vi "EG_G5210 ReadCh.vi"(0 "VISA Rsrc":refnum<visa-resource-name>="SR530", 1 "StatusByteRef":refnum<vi>, 5 "Channel":T1(ring), 7 "Autoscale":bool, 9 "Check Status":bool=TRUE, 11 "error in (no error)":errorcluster, 12 "Ask Correction":bool, 13 "ShowStatMess":bool=TRUE caption="Show Status Message") -> (2 "Sensitivity":u16(ring)=13 items=["100 nV", "300 nV", "1 µV", "3 µV", "10 µV", "30 µV", "100µV", "300 µV", "1 mV", "3 mV", "10 mV", "30 mV", "100 mV", "300 mV", "1 V", "3 V"], 3 "Status Byte":bool[](array[boolean]), 4 "Ressource VISA Out":refnum<visa-resource-name>="GPIB0::8::INSTR", 6 "Outputs":dbl[](array[numeric]), 8 "Outputs %":dbl[](array[numeric]), 10 "Warning":bool, 14 "Ask Correction Out":bool, 15 "error out":errorcluster)   [LabVIEW 2010]
uses:
  <userlib>/EG_G 5210 LIA/ReadChStates.ctl
  <userlib>/EG_G 5210 LIA/ReadFunctions.ctl
panel:
  out "Input Mode":u16(ring) items=["Current 10E8 A/V", "Current 10E6 A/V", "Voltage"]
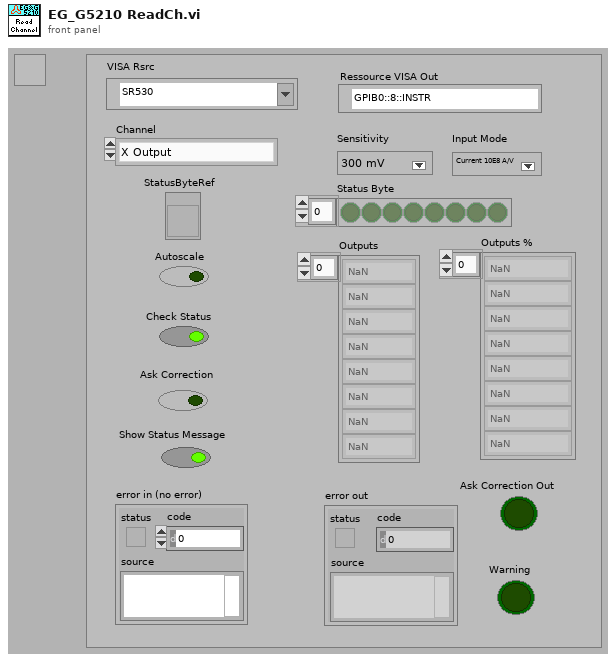
[diagram p1: front panel]
types:
  T1 = enum16{"X Output", "Y Output", "X and Y Output", "Mag", "Phase", "Mag & Phase", "X,Y,Mag & Phase", "Noise", "Aux In 1", "Aux In 2", "Aux In 3", "Aux In 4"}
  T2 = typedef "ReadChStates.ctl" = enum16{"Check Status", "Read Scale", "Read Ch"}
  T3 = typedef "ReadFunctions.ctl" = enum16{"Sensitivity", "Vernier Mode", "Main Filter", "Filter Mode", "Line Filter", "Ref Source", "Ref Mode", "Ref Phase", "Ref Frequency", "Output Filter", "Time Constant", "Dyn Reserve", "X Offset", "Y Offset", "Expand Mode", "Int Oscillator", "Oscillator Freq", "All params", "Overload Byte", "Trigger Mode", "Error"}
  T4 = typedef "LockInPar.ctl" = cluster{"Sensitivity":u16, "Vernier Mode":bool, "Vernier Value":i32, "Main Filter":u16, "Filter Freq (Hz)":dbl, "Filter Mode":u16, " Line Notch":u16, "Reference":u16, "Reference Mode":u16, "Ref Phase (°)":dbl, "Ref Freq (Hz)":dbl, "Output Filter":u16, "Time Constant":u16, "Dynamic Res.":u16, "X Offset":bool, "X Offset Val %":dbl, "Y Offset":bool, "Y Offset Val %":dbl, "Expand":bool, "Osc Amp. (mV rms)":i32, "Int Osc (Hz)":dbl, "Trigger Mode":u16, "Input Mode":u16, "Ovld Source":u16}
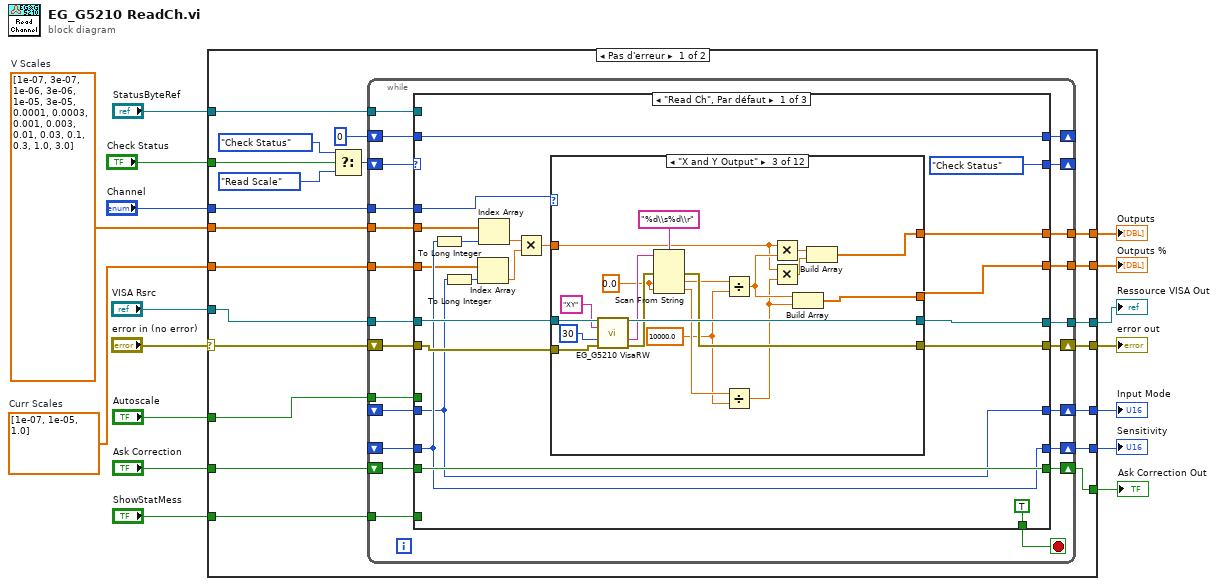
[diagram p0: block diagram]
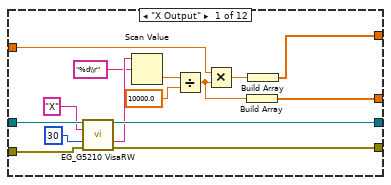
[diagram p2: hidden frame]
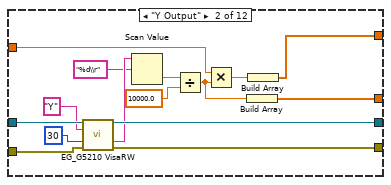
[diagram p3: hidden frame]
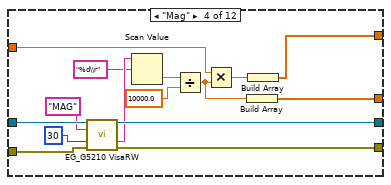
[diagram p4: hidden frame]
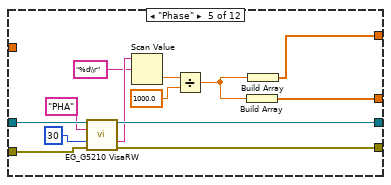
[diagram p5: hidden frame]
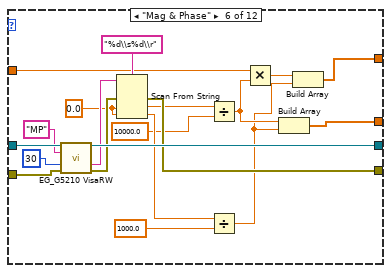
[diagram p6: hidden frame]
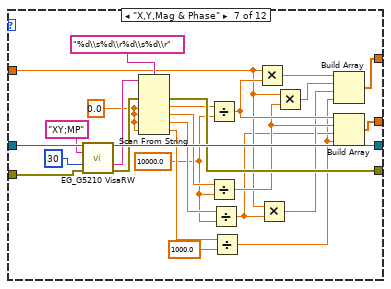
[diagram p7: hidden frame]
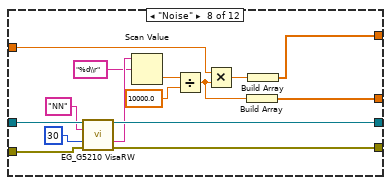
[diagram p8: hidden frame]
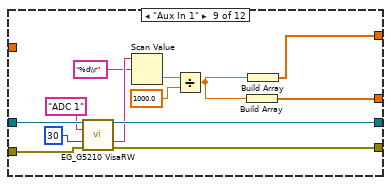
[diagram p9: hidden frame]
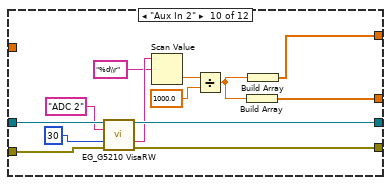
[diagram p10: hidden frame]
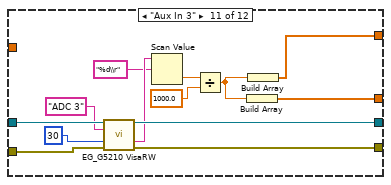
[diagram p11: hidden frame]
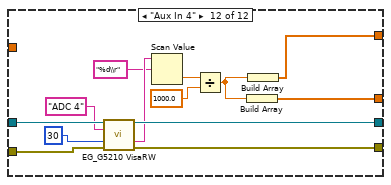
[diagram p12: hidden frame]
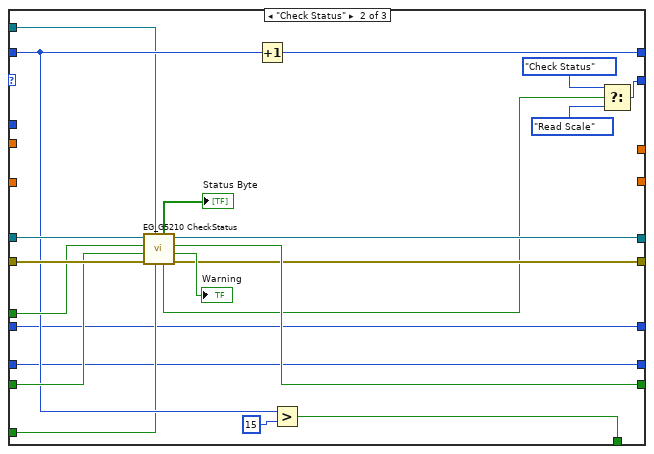
[diagram p13: hidden frame]
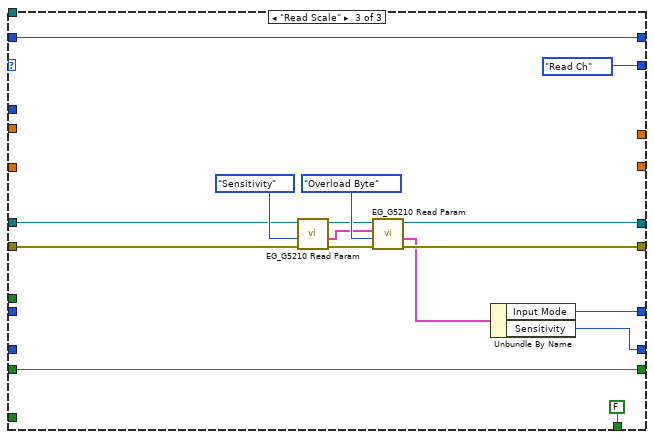
[diagram p14: hidden frame]
diagram:
  w1 = dbl[] [1e-07, 1e-05, 1.0]  # Curr Scales
  w8 = dbl[] [1e-07, 3e-07, 1e-06, 3e-06, 1e-05, 3e-05, 0.0001, 0.0003, 0.001, 0.003, 0.01, 0.03, 0.1, 0.3, 1.0, 3.0]  # V Scales
  n1 = case shown="Pas d'erreur" "error in (no error)" {
    selector: "error in (no error)" -> [w34 w311]
    tunnel: [w38 w311] -> w16
    tunnel: "Autoscale" -> [w37 _]
    tunnel: "Check Status" -> [w20 _]
    tunnel: "VISA Rsrc" -> [w35 w310]
    tunnel: "Ask Correction" -> [w33 _]
    tunnel: [w32 w310] -> w11
    tunnel: "StatusByteRef" -> [w31 _]
    tunnel: "ShowStatMess" -> [w30 _]
    tunnel: w8 -> [w29 _]
    tunnel: [w28 _] -> w7
    tunnel: [w27 _] -> w6
    tunnel: [w26 _] -> w5
    tunnel: "Channel" -> [w25 _]
    tunnel: [w24 _] -> w3
    tunnel: [w23 _] -> w2
    tunnel: w1 -> [w18 _]
    frame No Error {
      n2 = Select(t=ReadChStates."Check Status" ("Énum"), s=w20, f=ReadChStates."Read Scale" ("Énum")) -> (s? t:f=w19:T2)
      n3 = while {
        shift-right: [w57] -> _
        shift-left: w19 -> [w61]
        shift-right: [w59] -> w38
        shift-left: w34 -> [w60]
        tunnel: w37 -> [w56]
        tunnel: w25 -> [w55]
        shift-right: [w53] -> _
        shift-left: 0 ("timeout ms (488.2 global)") -> [w54]
        tunnel: w35 -> [w52]
        tunnel: [w50] -> w32
        tunnel: w31 -> [w49]
        tunnel: w30 -> [w48]
        tunnel: w29 -> [w47]
        shift-right: [w46] -> w28
        shift-left: _ -> [w43]
        shift-right: [w45] -> w27
        shift-left: _ -> [w40]
        shift-right: [w44] -> w26
        shift-left: w33 -> [w51]
        tunnel: [w42] -> w24
        tunnel: [w41] -> w23
        tunnel: w18 -> [w39]
        stop <- w58 stop-if-true
        n4 = case shown="\"Read Ch\", Par défaut" w61 {
          tunnel: w60 -> [w78 w293 w297]
          tunnel: [w79 w276 w304] -> w59
          tunnel: [TRUE w282 FALSE] -> w58
          tunnel: [ReadChStates."Check Status" ("Énum") w279 ReadChStates."Read Ch" ("Énum")] -> w57
          tunnel: w56 -> [_ w290 _]
          tunnel: w55 -> [w72 _ _]
          tunnel: w54 -> [w81 w286 w299]
          tunnel: [w81 w287 w299] -> w53
          tunnel: w52 -> [w77 w292 w296]
          tunnel: w51 -> [w74 w288 w295]
          tunnel: [w80 w277 w305] -> w50
          tunnel: w49 -> [_ w284 _]
          tunnel: w48 -> [_ w283 _]
          tunnel: w47 -> [w75 _ _]
          tunnel: [w69 w275 w301] -> w46
          tunnel: [w66 w274 w300] -> w45
          tunnel: [w74 w278 w295] -> w44
          tunnel: w43 -> [w69 w275 _]
          tunnel: [w71 _ _] -> w42
          tunnel: [w70 _ _] -> w41
          tunnel: w40 -> [w66 w274 _]
          tunnel: w39 -> [w67 _ _]
          frame "Read Ch", Default {
            n5 = To Long Integer(number=w69) -> (32bit integer=w73:i32)
            n6 = To Long Integer(number=w66) -> (32bit integer=w65:i32)
            n7 = Index Array(array=w67, index=w65) -> (element=w63:dbl)
            n8 = Index Array(array=w75, index=w73) -> (element=w64:dbl)
            n9 = Multiply(x=w64, y=w63) -> (x*y=w62:dbl)
            n10 = case shown="\"X and Y Output\"" w72 {
              tunnel: [w95 w110 w130 w145 w158 w178 w204 w219 w232 w245 w258 w271] -> w80
              tunnel: [w94 w109 w120 w144 w157 w168 w194 w218 w231 w244 w257 w270] -> w79
              tunnel: w78 -> [w93 w108 w129 w143 w156 w177 w203 w217 w230 w243 w256 w269]
              tunnel: w77 -> [w92 w107 w128 w142 w155 w176 w202 w216 w229 w242 w255 w268]
              tunnel: w62 -> [w86 w101 w112 w136 _ w162 w184 w210 _ _ _ _]
              tunnel: [w83 w98 w123 w133 w149 w171 w197 w207 w223 w236 w249 w262] -> w71
              tunnel: [w82 w97 w122 w132 w148 w170 w196 w206 w222 w235 w248 w261] -> w70
              frame "X Output" {
                n11 = call <userlib>:"EG_G5210 VisaRW.vi"("VISA Rsrc"=w92, "ChaineCom"="X", "Nbcaract"=u32 30, "error in (no error)"=w93) -> ("VISA Rsrc Out"=w95:refnum<visa-resource-name>, "ChaineRep"=w90:string, "error out"=w94:errorcluster)  [unwired: 8 in, 1 out]
                n12 = Scan Value(string=w90, format string="%d\\r" ("chaîne de format")) -> (value=w88:dbl)  [unwired: 1 in, 1 out]
                n13 = Divide(x=w88, y=10000.0) -> (x/y=w84:dbl)
                n14 = Multiply(x=w86, y=w84) -> (x*y=w85:dbl)
                n15 = Build Array(w84) -> (w82:dbl[])
                n16 = Build Array(w85) -> (w83:dbl[])
              }
              frame "Y Output" {
                n17 = call <userlib>:"EG_G5210 VisaRW.vi"("VISA Rsrc"=w107, "ChaineCom"="Y", "Nbcaract"=u32 30, "error in (no error)"=w108) -> ("VISA Rsrc Out"=w110:refnum<visa-resource-name>, "ChaineRep"=w105:string, "error out"=w109:errorcluster)  [unwired: 8 in, 1 out]
                n18 = Scan Value(string=w105, format string="%d\\r" ("chaîne de format")) -> (value=w103:dbl)  [unwired: 1 in, 1 out]
                n19 = Divide(x=w103, y=10000.0) -> (x/y=w99:dbl)
                n20 = Multiply(x=w101, y=w99) -> (x*y=w100:dbl)
                n21 = Build Array(w99) -> (w97:dbl[])
                n22 = Build Array(w100) -> (w98:dbl[])
              }
              frame "X and Y Output" {
                w117 = 0.0
                w115 = 10000.0 ("y")
                n23 = call <userlib>:"EG_G5210 VisaRW.vi"("VISA Rsrc"=w128, "ChaineCom"="XY", "Nbcaract"=u32 30, "error in (no error)"=w129) -> ("VISA Rsrc Out"=w130:refnum<visa-resource-name>, "ChaineRep"=w126:string, "error out"=w121:errorcluster)  [unwired: 8 in, 1 out]
                n24 = Scan From String(format string="%d\\s%d\\r" ("chaîne de format"), input string=w126, error in=w121, default 1=w117, default 2=w117) -> (error out=w120:errorcluster, output 1=w119:dbl, output 2=w116:dbl)  [unwired: 1 in, 2 out]
                n25 = Divide(x=w119, y=w115) -> (x/y=w124:dbl)
                n26 = Divide(x=w116, y=w115) -> (x/y=w113:dbl)
                n27 = Multiply(x=w112, y=w124) -> (x*y=w125:dbl)
                n28 = Multiply(x=w112, y=w113) -> (x*y=w114:dbl)
                n29 = Build Array(w124, w113) -> (w122:dbl[])
                n30 = Build Array(w125, w114) -> (w123:dbl[])
              }
              frame "Mag" {
                n31 = call <userlib>:"EG_G5210 VisaRW.vi"("VISA Rsrc"=w142, "ChaineCom"="MAG", "Nbcaract"=u32 30, "error in (no error)"=w143) -> ("VISA Rsrc Out"=w145:refnum<visa-resource-name>, "ChaineRep"=w140:string, "error out"=w144:errorcluster)  [unwired: 8 in, 1 out]
                n32 = Scan Value(string=w140, format string="%d\\r" ("chaîne de format")) -> (value=w138:dbl)  [unwired: 1 in, 1 out]
                n33 = Divide(x=w138, y=10000.0) -> (x/y=w134:dbl)
                n34 = Multiply(x=w136, y=w134) -> (x*y=w135:dbl)
                n35 = Build Array(w134) -> (w132:dbl[])
                n36 = Build Array(w135) -> (w133:dbl[])
              }
              frame "Phase" {
                n37 = call <userlib>:"EG_G5210 VisaRW.vi"("VISA Rsrc"=w155, "ChaineCom"="PHA", "Nbcaract"=u32 30, "error in (no error)"=w156) -> ("VISA Rsrc Out"=w158:refnum<visa-resource-name>, "ChaineRep"=w153:string, "error out"=w157:errorcluster)  [unwired: 8 in, 1 out]
                n38 = Scan Value(string=w153, format string="%d\\r" ("chaîne de format")) -> (value=w151:dbl)  [unwired: 1 in, 1 out]
                n39 = Divide(x=w151, y=1000.0) -> (x/y=w147:dbl)
                n40 = Build Array(w147) -> (w148:dbl[])
                n41 = Build Array(w147) -> (w149:dbl[])
              }
              frame "Mag & Phase" {
                w165 = 0.0
                n42 = call <userlib>:"EG_G5210 VisaRW.vi"("VISA Rsrc"=w176, "ChaineCom"="MP", "Nbcaract"=u32 30, "error in (no error)"=w177) -> ("VISA Rsrc Out"=w178:refnum<visa-resource-name>, "ChaineRep"=w174:string, "error out"=w169:errorcluster)  [unwired: 8 in, 1 out]
                n43 = Scan From String(format string="%d\\s%d\\r" ("chaîne de format"), input string=w174, error in=w169, default 1=w165, default 2=w165) -> (error out=w168:errorcluster, output 1=w167:dbl, output 2=w164:dbl)  [unwired: 1 in, 2 out]
                n44 = Divide(x=w167, y=10000.0) -> (x/y=w172:dbl)
                n45 = Divide(x=w164, y=1000.0) -> (x/y=w161:dbl)
                n46 = Multiply(x=w162, y=w172) -> (x*y=w173:dbl)
                n47 = Build Array(w172, w161) -> (w170:dbl[])
                n48 = Build Array(w173, w161) -> (w171:dbl[])
              }
              frame "X,Y,Mag & Phase" {
                w188 = 0.0
                w185 = 10000.0 ("y")
                n49 = call <userlib>:"EG_G5210 VisaRW.vi"("VISA Rsrc"=w202, "ChaineCom"="XY;MP", "Nbcaract"=u32 30, "error in (no error)"=w203) -> ("VISA Rsrc Out"=w204:refnum<visa-resource-name>, "ChaineRep"=w200:string, "error out"=w195:errorcluster)  [unwired: 8 in, 1 out]
                n50 = Scan From String(format string="%d\\s%d\\r%d\\s%d\\r" ("chaîne de format"), input string=w200, error in=w195, default 1=w188, default 2=w188, default 3=w188, default 4=w188) -> (error out=w194:errorcluster, output 1=w193:dbl, output 2=w191:dbl, output 3=w187:dbl, output 4=w186:dbl)  [unwired: 1 in, 2 out]
                n51 = Divide(x=w193, y=w185) -> (x/y=w198:dbl)
                n52 = Divide(x=w191, y=w185) -> (x/y=w189:dbl)
                n53 = Divide(x=w187, y=w185) -> (x/y=w182:dbl)
                n54 = Divide(x=w186, y=1000.0) -> (x/y=w181:dbl)
                n55 = Multiply(x=w184, y=w198) -> (x*y=w199:dbl)
                n56 = Multiply(x=w184, y=w182) -> (x*y=w183:dbl)
                n57 = Multiply(x=w184, y=w189) -> (x*y=w190:dbl)
                n58 = Build Array(w199, w190, w183, w181) -> (w197:dbl[])
                n59 = Build Array(w198, w189, w182, w181) -> (w196:dbl[])
              }
              frame "Noise" {
                n60 = call <userlib>:"EG_G5210 VisaRW.vi"("VISA Rsrc"=w216, "ChaineCom"="NN", "Nbcaract"=u32 30, "error in (no error)"=w217) -> ("VISA Rsrc Out"=w219:refnum<visa-resource-name>, "ChaineRep"=w214:string, "error out"=w218:errorcluster)  [unwired: 8 in, 1 out]
                n61 = Scan Value(string=w214, format string="%d\\r" ("chaîne de format")) -> (value=w212:dbl)  [unwired: 1 in, 1 out]
                n62 = Divide(x=w212, y=10000.0) -> (x/y=w208:dbl)
                n63 = Multiply(x=w210, y=w208) -> (x*y=w209:dbl)
                n64 = Build Array(w208) -> (w206:dbl[])
                n65 = Build Array(w209) -> (w207:dbl[])
              }
              frame "Aux In 1" {
                n66 = call <userlib>:"EG_G5210 VisaRW.vi"("VISA Rsrc"=w229, "ChaineCom"="ADC 1", "Nbcaract"=u32 30, "error in (no error)"=w230) -> ("VISA Rsrc Out"=w232:refnum<visa-resource-name>, "ChaineRep"=w227:string, "error out"=w231:errorcluster)  [unwired: 8 in, 1 out]
                n67 = Scan Value(string=w227, format string="%d\\r" ("chaîne de format")) -> (value=w225:dbl)  [unwired: 1 in, 1 out]
                n68 = Divide(x=w225, y=1000.0) -> (x/y=w221:dbl)
                n69 = Build Array(w221) -> (w222:dbl[])
                n70 = Build Array(w221) -> (w223:dbl[])
              }
              frame "Aux In 2" {
                n71 = call <userlib>:"EG_G5210 VisaRW.vi"("VISA Rsrc"=w242, "ChaineCom"="ADC 2", "Nbcaract"=u32 30, "error in (no error)"=w243) -> ("VISA Rsrc Out"=w245:refnum<visa-resource-name>, "ChaineRep"=w240:string, "error out"=w244:errorcluster)  [unwired: 8 in, 1 out]
                n72 = Scan Value(string=w240, format string="%d\\r" ("chaîne de format")) -> (value=w238:dbl)  [unwired: 1 in, 1 out]
                n73 = Divide(x=w238, y=1000.0) -> (x/y=w234:dbl)
                n74 = Build Array(w234) -> (w235:dbl[])
                n75 = Build Array(w234) -> (w236:dbl[])
              }
              frame "Aux In 3" {
                n76 = call <userlib>:"EG_G5210 VisaRW.vi"("VISA Rsrc"=w255, "ChaineCom"="ADC 3", "Nbcaract"=u32 30, "error in (no error)"=w256) -> ("VISA Rsrc Out"=w258:refnum<visa-resource-name>, "ChaineRep"=w253:string, "error out"=w257:errorcluster)  [unwired: 8 in, 1 out]
                n77 = Scan Value(string=w253, format string="%d\\r" ("chaîne de format")) -> (value=w251:dbl)  [unwired: 1 in, 1 out]
                n78 = Divide(x=w251, y=1000.0) -> (x/y=w247:dbl)
                n79 = Build Array(w247) -> (w248:dbl[])
                n80 = Build Array(w247) -> (w249:dbl[])
              }
              frame "Aux In 4" {
                n81 = call <userlib>:"EG_G5210 VisaRW.vi"("VISA Rsrc"=w268, "ChaineCom"="ADC 4", "Nbcaract"=u32 30, "error in (no error)"=w269) -> ("VISA Rsrc Out"=w271:refnum<visa-resource-name>, "ChaineRep"=w266:string, "error out"=w270:errorcluster)  [unwired: 8 in, 1 out]
                n82 = Scan Value(string=w266, format string="%d\\r" ("chaîne de format")) -> (value=w264:dbl)  [unwired: 1 in, 1 out]
                n83 = Divide(x=w264, y=1000.0) -> (x/y=w260:dbl)
                n84 = Build Array(w260) -> (w261:dbl[])
                n85 = Build Array(w260) -> (w262:dbl[])
              }
            }
          }
          frame "Check Status" {
            n86 = call <userlib>:"EG_G5210 CheckStatus.vi"("ShowStatMess"=w283, "StatusByteRef"=w284, "error in (no error)"=w293, "Ask Correction"=w288, "Autoscale"=w290, "Ressource VISA In"=w292) -> ("error out"=w276:errorcluster, "Warning"=→"Warning":bool, "Ask Correction Out"=w278:bool, "Ressource VISA Out"=w277:refnum<visa-resource-name>, "Reprise"=w273:bool, "Status Byte"=→"Status Byte":bool[])
            n87 = Increment(x=w286) -> (x+1=w287:i32)
            n88 = Greater?(x=w286, y=15) -> (0:w282:bool)
            n89 = Select(t=ReadChStates."Check Status" ("Énum"), s=w273, f=ReadChStates."Read Scale" ("Énum")) -> (s? t:f=w279:T2)
          }
          frame "Read Scale" {
            n90 = call <userlib>:"EG_G5210 Read Param.vi"("error in (no error)"=w297, "Énum"=ReadFunctions."Sensitivity", "Ressource VISA"=w296) -> ("error out"=w307:errorcluster, "LockInPar"=w303:T4, "Ressource VISA Out"=w306:refnum<visa-resource-name>)  [unwired: 5 in, 1 out]
            n91 = call <userlib>:"EG_G5210 Read Param.vi"("error in (no error)"=w307, "Énum"=ReadFunctions."Overload Byte", "LockInPar In"=w303, "Ressource VISA"=w306) -> ("error out"=w304:errorcluster, "LockInPar"=w302:T4, "Ressource VISA Out"=w305:refnum<visa-resource-name>)  [unwired: 4 in, 1 out]
            n92 = Unbundle By Name(w302) -> ("Input Mode"=w300:u16, "Sensitivity"=w301:u16)
          }
        }
      }
    }
    frame Error {
    }
  }
  "error out" <- w16
  "Ressource VISA Out" <- w11
  "Sensitivity" <- w7
  "Input Mode" <- w6
  "Outputs" <- w3
  "Outputs %" <- w2
  "Ask Correction Out" <- w5
